vi "JSON Array Probe.vi"(11 "JSON Array In":refnum<class "JSON Array.lvclass">) -> (2 "Value String":string, 3 "Boolean":bool)   [LabVIEW 2020, in "Library Commun.lvlib" / "JSON Array.lvclass"]
uses:
  JSON Array.lvclass
panel:
  out "JSON":string
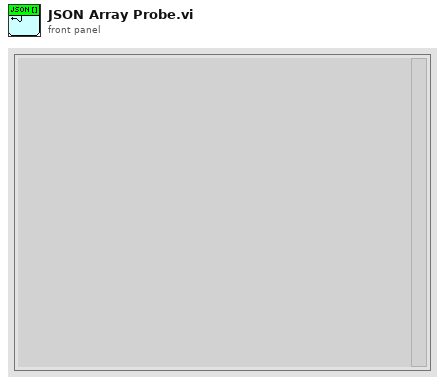
[diagram p1: front panel]
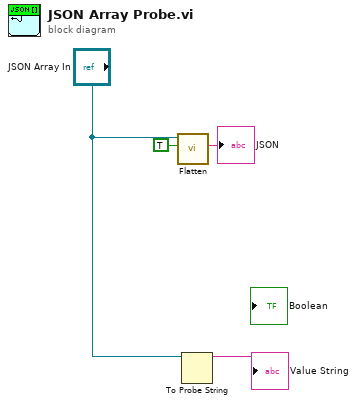
[diagram p0: block diagram]
diagram:
  n1 = call-dynamic "Flatten.vi"("Pretty Print?"=TRUE, "JSON Array in"="JSON Array In") -> ("<JSON>"=→"JSON":string)  [unwired: 8 in, 1 out]
  n2 = To Probe String(7:"JSON Array In") -> (3:→"Value String":string)  [unwired: 2 in, 1 out]
